vi "Update WPC Stats File v2.vi"(11 "file path (use dialog)":path=path "C:/Users/manma/Google Drive/WPC Stat Scrape/Data/WPC Stats.bin") -> (0 "error out":errorcluster, 1 "redacted?":bool, 2 "File Updated?":bool, 3 "Full WPC Stats":T1[][](array[typedef]) {"Date Updated" format="%<%m/%d/%Y>T"})   [LabVIEW 2021]
uses:
  WPC Player and Financial Stats.ctl
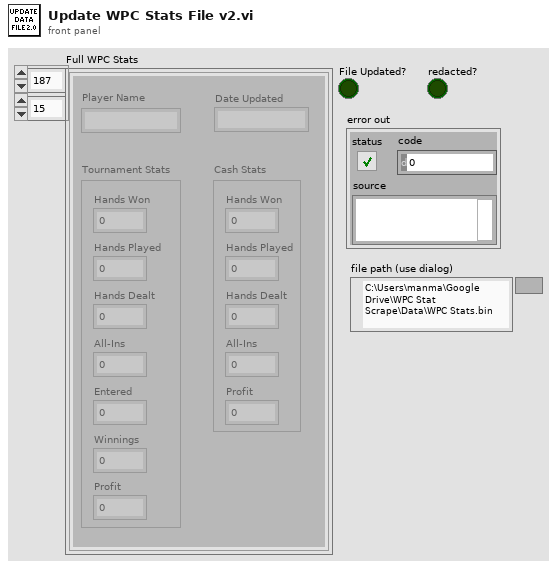
[diagram p1: front panel]
types:
  T1 = typedef "WPC Player and Financial Stats.ctl" = cluster{"Player Name":string, "Date Updated":timestamp, "Tournament Stats":cluster{"Hands Won":i32, "Hands Played":i32, "Hands Dealt":i32, "All-Ins":i32, "Entered":i32, "Winnings":dbl, "Profit":dbl}, "Cash Stats":cluster{"Hands Won":i32, "Hands Played":i32, "Hands Dealt":i32, "All-Ins":i32, "Profit":dbl}}
  T2 = enum16{"open", "replace", "create", "open or create", "replace or create", "replace or create with confirmation"}
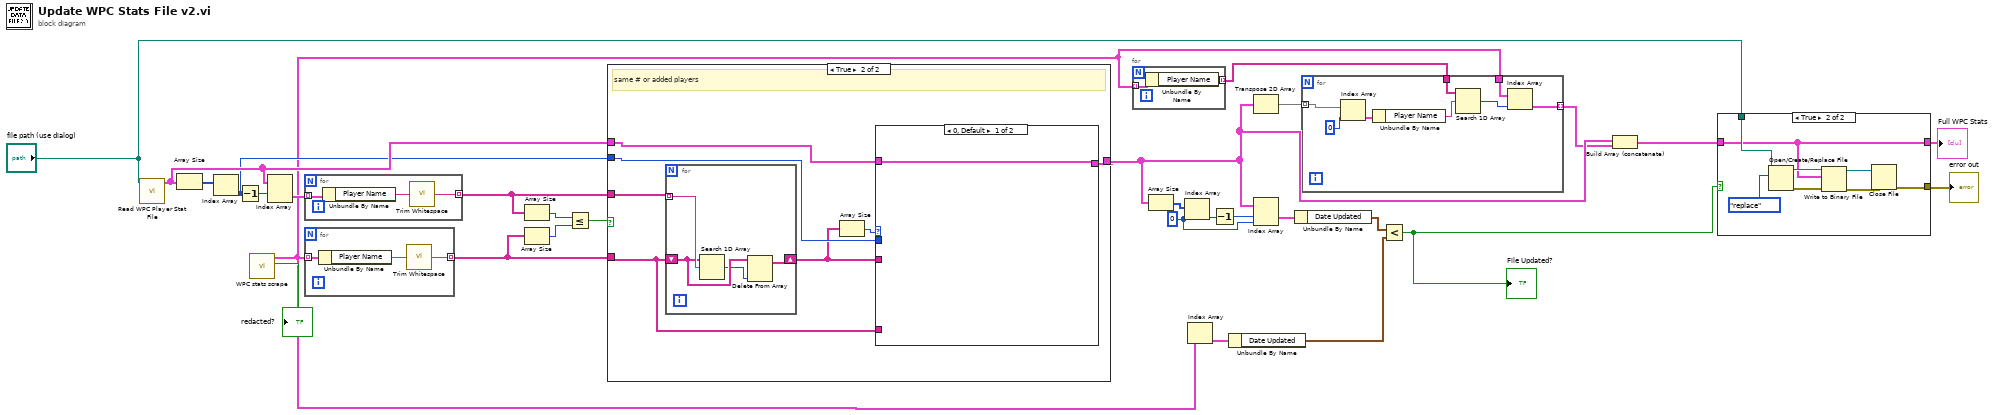
[diagram p0: block diagram]
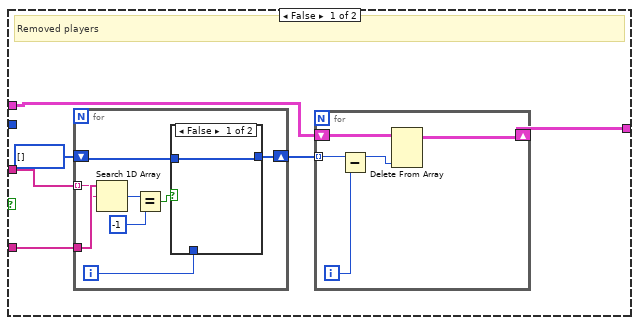
[diagram p2: hidden frame]
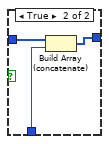
[diagram p3: hidden frame]
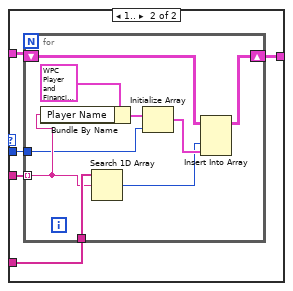
[diagram p4: hidden frame]
diagram:
  w22 = 0 ("index")
  n1 = call "Read WPC Player Stat File.vi"("file path (use dialog)"="file path (use dialog)") -> ("Full WPC Stats"=w27:T1[][])  [unwired: 8 in, 2 out]
  n2 = Array Size(array=w27) -> (size(s)=w29:i32[])
  n3 = Index Array(array=w29) -> (element=w16:i32)  [unwired: 1 in]
  n4 = Decrement(x=w16) -> (x-1=w26:i32)
  n5 = call "WPC stats scrape.vi"() -> ("redacted?"=→"redacted?":bool, "WPC Player Stats"=w7:T1[])  [unwired: 10 in]
  n6 = Index Array(array=w27, index (row)=w26) -> (element=w28:T1[])  [unwired: 1 in]
  n7 = for {
    tunnel: w28 -> [w32] mode=indexing
    tunnel: [w30] -> w14 mode=indexing
    n8 = Unbundle By Name(w32) -> ("Player Name"=w31:string)
    n9 = call <vilib>:"Trim Whitespace.vi"("string"=w31) -> ("trimmed string"=w30:string)  [unwired: 1 in]
  }
  n10 = for {
    tunnel: w7 -> [w35] mode=indexing
    tunnel: [w33] -> w13 mode=indexing
    n11 = Unbundle By Name(w35) -> ("Player Name"=w34:string)
    n12 = call <vilib>:"Trim Whitespace.vi"("string"=w34) -> ("trimmed string"=w33:string)  [unwired: 1 in]
  }
  n13 = Array Size(array=w14) -> (size(s)=w12:i32)
  n14 = Array Size(array=w13) -> (size(s)=w11:i32)
  n15 = Less Or Equal?(x=w12, y=w11) -> (x <= y?=w10:bool)
  n16 = case shown="True" w10 {
    tunnel: w14 -> [w40 w61]
    tunnel: w27 -> [w37 w65]
    tunnel: w13 -> [w41 w62]
    tunnel: w16 -> [_ w64]
    tunnel: [w36 w63] -> w5
    frame False {
      # "Removed players"
      n17 = for {
        tunnel: w41 -> [w48]
        tunnel: w40 -> [w47] mode=indexing
        shift-right: [w50] -> w38
        shift-left: i32[] [] -> [w51]
        i -> [w52]
        n18 = Search 1D Array(1D array=w48, element=w47) -> (index of element=w49:i32)  [unwired: 1 in]
        n19 = Equal?(x=w49, y=-1) -> (x = y?=w53:bool)
        n20 = case shown="False" w53 {
          tunnel: w52 -> [_ w58]
          tunnel: w51 -> [w55 w57]
          tunnel: [w55 w56] -> w50
          frame False {
          }
          frame True {
            n21 = Build Array (concatenate)(w57, w58) -> (w56:i32[])
          }
        }
      }
      n22 = for {
        tunnel: w38 -> [w43] mode=indexing
        shift-right: [w45] -> w36
        shift-left: w37 -> [w46]
        i -> [w42]
        n23 = Subtract(x=w43, y=w42) -> (x-y=w44:i32)
        n24 = Delete From Array(array=w46, index (col)=w44) -> (array with subset deleted=w45:T1[][])  [unwired: 2 in, 1 out]
      }
    }
    frame True {
      # "same # or added players"
      n25 = for {
        tunnel: w61 -> [w84] mode=indexing
        shift-right: [w82] -> w59
        shift-left: w62 -> [w83]
        n26 = Search 1D Array(1D array=w83, element=w84) -> (index of element=w81:i32)  [unwired: 1 in]
        n27 = Delete From Array(array=w83, index=w81) -> (array with subset deleted=w82:string[])  [unwired: 1 in, 1 out]
      }
      n28 = Array Size(array=w59) -> (size(s)=w60:i32)
      n29 = case shown="0, Default" w60 {
        tunnel: w65 -> [w66 w71]
        tunnel: w64 -> [_ w70]
        tunnel: [w66 w69] -> w63
        tunnel: w62 -> [_ w68]
        tunnel: w59 -> [_ w67]
        frame 0, Default {
        }
        frame 1.. {
          n30 = for {
            tunnel: w67 -> [w78] mode=indexing
            tunnel: w68 -> [w80]
            tunnel: w70 -> [w76]
            shift-right: [w74] -> w69
            shift-left: w71 -> [w79]
            n31 = Bundle By Name(cluster=T1 {"Player Name"="", "Date Updated"=timestamp(0 s since 1904-01-01), "Tournament Stats"={"Hands Won"=0, "Hands Played"=0, "Hands Dealt"=0, "All-Ins"=0, "Entered"=0, "Winnings"=0.0, "Profit"=0.0}, "Cash Stats"={"Hands Won"=0, "Hands Played"=0, "Hands Dealt"=0, "All-Ins"=0, "Profit"=0.0}} ("Full WPC Stats"), "Player Name"=w78) -> (w77:T1)
            n32 = Search 1D Array(1D array=w80, element=w78) -> (index of element=w73:i32)  [unwired: 1 in]
            n33 = Initialize Array(w77, w76) -> (w75:T1[])
            n34 = Insert Into Array(array=w79, index (col)=w73, new element=w75) -> (w74:T1[][])  [unwired: 1 in]
          }
        }
      }
    }
  }
  n35 = for {
    tunnel: w7 -> [w86] mode=indexing
    tunnel: [w85] -> w8 mode=indexing
    n36 = Unbundle By Name(w86) -> ("Player Name"=w85:string)
  }
  n37 = Array Size(array=w5) -> (size(s)=w25:i32[])
  n38 = Index Array(array=w25, index=w22) -> (element=w24:i32)
  n39 = Index Array(array=w7) -> (element=w20:T1)  [unwired: 1 in]
  n40 = Decrement(x=w24) -> (x-1=w23:i32)
  n41 = Unbundle By Name(w20) -> ("Date Updated"=w18:timestamp)
  n42 = Transpose 2D Array(2D array=w5) -> (transposed array=w6:T1[][])
  n43 = Index Array(array=w5, index (row)=w23, index (col)=w22) -> (element=w21:T1)
  n44 = Unbundle By Name(w21) -> ("Date Updated"=w19:timestamp)
  n45 = for {
    tunnel: w6 -> [w88] mode=indexing
    tunnel: w8 -> [w92]
    tunnel: w7 -> [w90]
    tunnel: [w87] -> w4 mode=indexing
    n46 = Index Array(array=w88, index=0) -> (element=w93:T1)
    n47 = Unbundle By Name(w93) -> ("Player Name"=w91:string)
    n48 = Search 1D Array(1D array=w92, element=w91) -> (index of element=w89:i32)  [unwired: 1 in]
    n49 = Index Array(array=w90, index=w89) -> (element=w87:T1)
  }
  n50 = Less?(x=w19, y=w18) -> (x < y?=w1:bool)
  "File Updated?" <- w1
  n51 = Build Array (concatenate)(w5, w4) -> (w3:T1[][])
  n52 = case shown="True" w1 {
    tunnel: [_ w103] -> w17
    tunnel: "file path (use dialog)" -> [_ w102]
    tunnel: w3 -> [w95 w96]
    tunnel: [w95 w96] -> w2
    frame False {
    }
    frame True {
      n53 = Open/Create/Replace File(file path (use dialog)=w102, operation (0:open)=T2."replace") -> (refnum out=w99:refnum<file>, error out=w100:errorcluster)  [unwired: 4 in, 1 out]
      n54 = Write to Binary File(file (use dialog)=w99, data=w96, error in=w100) -> (refnum out=w98:refnum<file>, error out=w97:errorcluster)  [unwired: 3 in, 1 out]
      n55 = Close File(refnum=w98, error in=w97) -> (error out=w103:errorcluster)  [unwired: 1 out]
    }
  }
  "error out" <- w17
  "Full WPC Stats" <- w2
